vi "Test Is States Constant - String Constant Outside JKI SM.vi"(8 "error in (no error)":errorcluster) -> (0 "error out":errorcluster)   [LabVIEW 2020, in "TEST JKI State Machine API.lvlib"]
uses:
  TEST JKI State Machine API.lvlib
  source/JKI State Machine API.lvlib
  <vilib>/addons/_JKI Toolkits/Caraya/classes/Test/Test.lvclass
  <vilib>/addons/_JKI Toolkits/Caraya/classes/Assert/Assert.lvclass
  source/JKI SM/JKI SM.lvclass
panel:
  out "Structure Found in":refnum<vi>
  out "Found JKI SMs?":bool
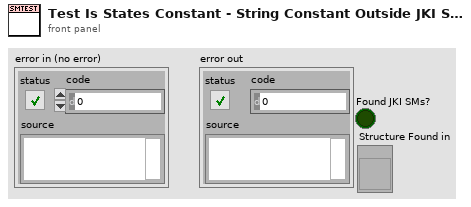
[diagram p1: front panel]
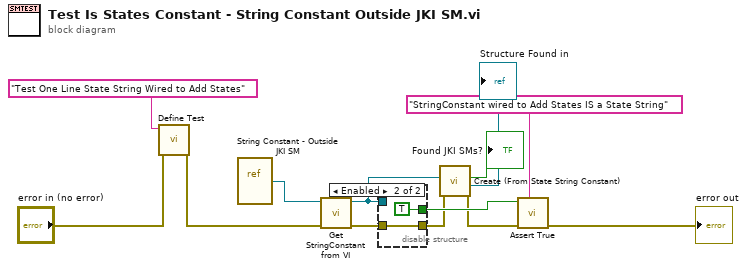
[diagram p0: block diagram]
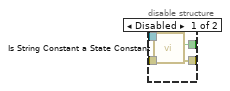
[diagram p2: hidden frame]
diagram:
  n1 = call <vilib>:"Define Test.vi"("error in (no error)"="error in (no error)", "Label (VI Title)"="Test One Line State String Wired to Add States") -> ("error out"=w12:errorcluster)  [unwired: 8 in, 1 out]
  n2 = vi-ref "String Constant - Outside JKI SM.vi"() -> (w9:refnum<vi>)
  n3 = call "Get StringConstant from VI.vi"("error in (no error)"=w12, "VI in"=w9) -> ("error out"=w8:errorcluster, "StringConstant out"=w5:refnum<vi>)  [unwired: 8 in]
  n4 = disable-structure shown="Enabled" {
    disable-tunnel: [w17 TRUE ("True?")] -> w13
    disable-tunnel: w8 -> [w16 w19]
    disable-tunnel: w5 -> [w15 _]
    disable-tunnel: [w14 w19] -> w4
    frame Disabled {
      n5 = call "Is String Constant a State Constant.vi"("error in (no error)"=w16, "GObj Refnum"=w15) -> ("error out"=w14:errorcluster, "Is States Constant"=w17:bool)  [unwired: 7 in, 1 out]
    }
    frame Enabled {
    }
  }
  n6 = call "Create (From State String Constant).vi"("error in (no error)"=w4, "State String Constant"=w5) -> ("error out"=w3:errorcluster, "Structure Found in"=→"Structure Found in":refnum<vi>, "Found JKI SMs?"=→"Found JKI SMs?":bool)  [unwired: 6 in, 1 out]
  n7 = call <vilib>:"Assert True.vi"("Label"="StringConstant wired to Add States IS a State String", "error in (no error)"=w3, "True?"=w13) -> ("error out"=→"error out":errorcluster)  [unwired: 7 in, 1 out]
